vi "Initialize.vi"(8 "error in (no error)":errorcluster, 11 "UDP Buffer Converter in":refnum<class "UDP Buffer Converter.lvclass">) -> (0 "error out":errorcluster, 3 "UDP Buffer Converter out":refnum<class "UDP Buffer Converter.lvclass">)   [LabVIEW 2017, in "UDP.lvlib" / "UDP Buffer Converter.lvclass"]
uses:
  UDP Buffer Converter.lvclass
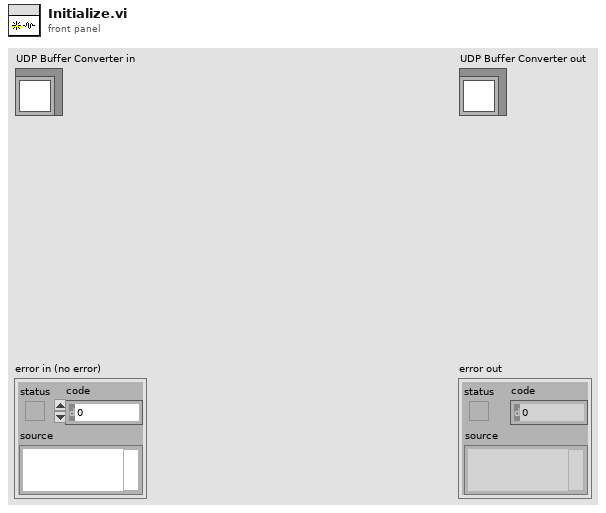
[diagram p1: front panel]
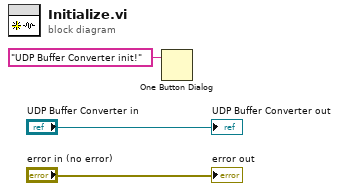
[diagram p0: block diagram]
diagram:
  n1 = One Button Dialog(message="UDP Buffer Converter init!") -> ()  [unwired: 1 in, 1 out]
  "error out" <- "error in (no error)"
  "UDP Buffer Converter out" <- "UDP Buffer Converter in"
